vi "WindowPosition.vi"(4 "Komunikat":refnum<vi>, 6 "WindowHandler":refnum<vi>, 8 "error in (no error)":errorcluster, 9 "STOP":refnum<vi>, 10 "Tab":refnum<vi>, 11 "VI in":refnum<vi>) -> (0 "error out":errorcluster)   [LabVIEW 2019]
uses:
  <vilib>/Utility/miscctls.llb/LVRectTypeDef.ctl
  <vilib>/Utility/miscctls.llb/LVPointTypeDef.ctl
  <vilib>/Utility/miscctls.llb/LVBoundsTypeDef.ctl
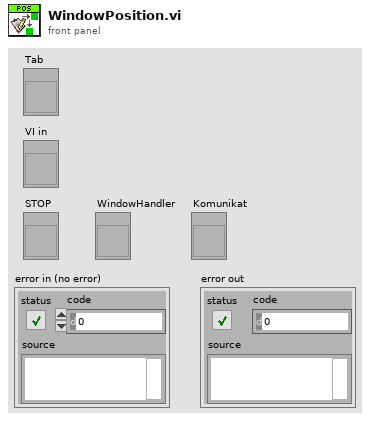
[diagram p1: front panel]
types:
  T1 = typedef "LVBoundsTypeDef.ctl" = cluster{"Width":u32, "Height":u32}
  T2 = typedef "LVPointTypeDef.ctl" = cluster{"Horizontal":i16, "Vertical":i16}
  T3 = typedef "LVRectTypeDef.ctl" = cluster{"Left":i16, "Top":i16, "Right":i16, "Bottom":i16}
  T4 = cluster{"Left":dbl, "Top":dbl, "Right":dbl, "Bottom":dbl}
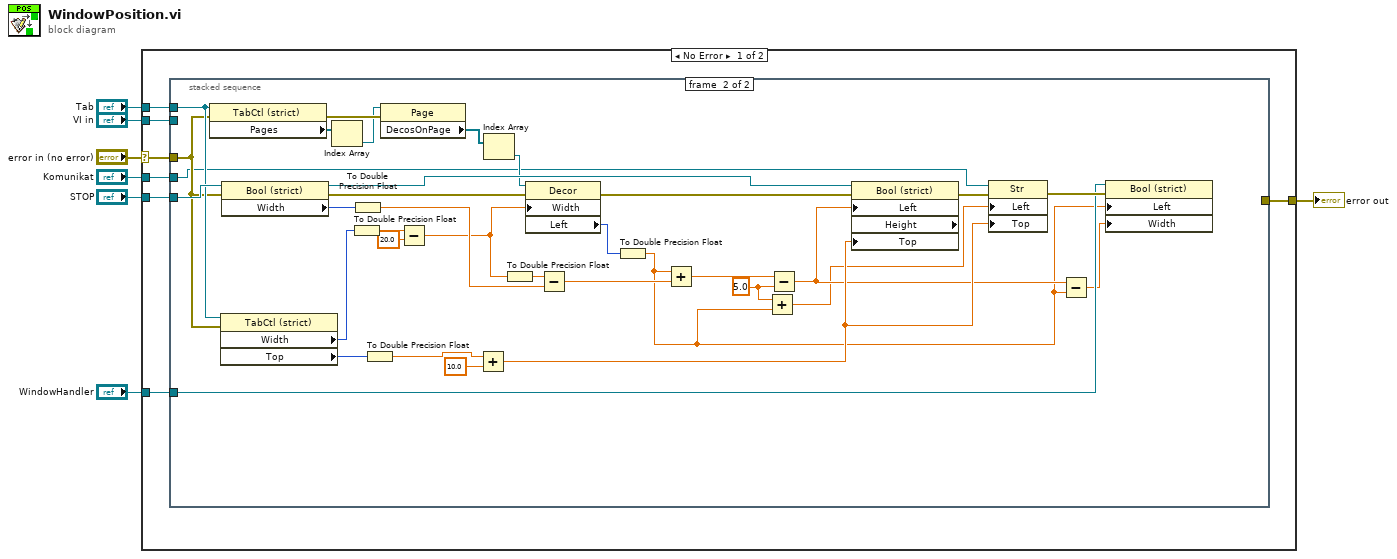
[diagram p0: block diagram]
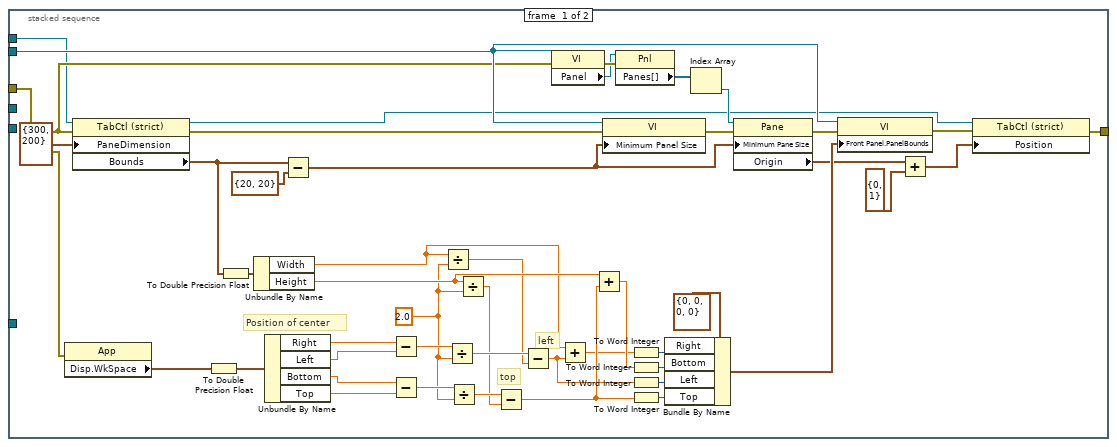
[diagram p2: hidden frame]
diagram:
  n1 = case shown="No Error" "error in (no error)" {
    selector: "error in (no error)" -> [w11 w95]
    tunnel: [w14 w95] -> w7
    tunnel: "Tab" -> [w13 _]
    tunnel: "VI in" -> [w12 _]
    tunnel: "STOP" -> [w10 _]
    tunnel: "Komunikat" -> [w9 _]
    tunnel: "WindowHandler" -> [w8 _]
    frame No Error {
      n2 = stacked-sequence {
        tunnel: [w60 _] -> w14
        tunnel: w13 -> [w17 w85]
        tunnel: w12 -> [w28 _]
        tunnel: w11 -> [w20 w84]
        tunnel: w10 -> [_ w86]
        tunnel: w9 -> [_ w82]
        tunnel: w8 -> [_ w65]
        frame #0 {
          w35 = 2.0
          # "Position of center"
          # "left"
          # "top"
          n3 = property class="App"(error in=w20) -> ("Disp.WkSpace"=w22:T3)  [unwired: 1 in, 2 out]
          n4 = property class="TabCtl (strict)"(reference=w17, error in=w20, "PaneDimension"=T1 {"Width"=300, "Height"=200} ("Tab Control Pane Dimension")) -> (reference out=w19:refnum<vi>, error out=w18:errorcluster, "Bounds"=w15:T1)
          n5 = To Double Precision Float(number=w22) -> (double precision float=w46:T4)
          n6 = To Double Precision Float(number=w15) -> (double precision float=w52:cluster{"Width":dbl, "Height":dbl})
          n7 = Unbundle By Name(w52) -> ("Width"=w34:dbl, "Height"=w54:dbl)
          n8 = Unbundle By Name(w46) -> ("Right"=w42:dbl, "Left"=w43:dbl, "Bottom"=w44:dbl, "Top"=w45:dbl)
          n9 = Subtract(x=w15, y=T2 {"Horizontal"=20, "Vertical"=20} ("Minimum Pane Size")) -> (x-y=w59:T1)
          n10 = Subtract(x=w42, y=w43) -> (x-y=w47:dbl)
          n11 = Subtract(x=w44, y=w45) -> (x-y=w48:dbl)
          n12 = Divide(x=w34, y=w35) -> (x/y=w33:dbl)
          n13 = Divide(x=w47, y=w35) -> (x/y=w36:dbl)
          n14 = Divide(x=w48, y=w35) -> (x/y=w37:dbl)
          n15 = Divide(x=w54, y=w35) -> (x/y=w32:dbl)
          n16 = Subtract(x=w37, y=w32) -> (x-y=w41:dbl)
          n17 = Subtract(x=w36, y=w33) -> (x-y=w40:dbl)
          n18 = property class="VI"(reference=w28, error in=w20) -> (error out=w57:errorcluster, "Panel"=w55:refnum<vi>)  [unwired: 1 out]
          n19 = Add(x=w34, y=w40) -> (x+y=w38:dbl)
          n20 = Add(x=w54, y=w41) -> (x+y=w39:dbl)
          n21 = property class="VI"(reference=w28, error in=w18, "Minimum Panel Size"=w59) -> (error out=w30:errorcluster)  [unwired: 1 out]
          n22 = property class="Pnl"(reference=w55, error in=w57) -> ("Panes[]"=w56:refnum<vi>[])  [unwired: 2 out]
          n23 = To Word Integer(number=w38) -> (16bit integer=w49:i16)
          n24 = To Word Integer(number=w39) -> (16bit integer=w51:i16)
          n25 = To Word Integer(number=w40) -> (16bit integer=w50:i16)
          n26 = To Word Integer(number=w41) -> (16bit integer=w53:i16)
          n27 = Bundle By Name(cluster=T3 {"Left"=0, "Top"=0, "Right"=0, "Bottom"=0} ("Front Panel Window:Panel Bounds"), "Right"=w49, "Bottom"=w51, "Left"=w50, "Top"=w53) -> (w27:T3)
          n28 = Index Array(array=w56) -> (element=w58:refnum<vi>)  [unwired: 1 in]
          n29 = property class="Pane"(reference=w58, error in=w30, "Minimum Pane Size"=w59) -> (error out=w29:errorcluster, "Origin"=w26:T2)  [unwired: 1 out]
          n30 = property class="VI"(reference=w28, error in=w29, "Front Panel.PanelBounds"=w27) -> (error out=w24:errorcluster)  [unwired: 1 out]
          n31 = Add(x=w26, y=T2 {"Horizontal"=0, "Vertical"=1}) -> (x+y=w25:T2)
          n32 = property class="TabCtl (strict)"(reference=w19, error in=w24, "Position"=w25) -> (error out=w60:errorcluster)  [unwired: 1 out]
        }
        frame #1 {
          w79 = 5.0 ("y")
          n33 = property class="TabCtl (strict)"(reference=w85, error in=w84) -> (error out=w90:errorcluster, "Pages"=w89:refnum<vi>[])  [unwired: 1 out]
          n34 = property class="TabCtl (strict)"(reference=w85, error in=w84) -> ("Width"=w71:u32, "Top"=w72:i32)  [unwired: 2 out]
          n35 = property class="Bool (strict)"(reference=w86, error in=w84) -> (reference out=w93:refnum<vi>, error out=w94:errorcluster, "Width"=w77:u32)
          n36 = Index Array(array=w89) -> (element=w88:refnum<vi>)  [unwired: 1 in]
          n37 = To Double Precision Float(number=w71) -> (double precision float=w70:dbl)
          n38 = To Double Precision Float(number=w77) -> (double precision float=w76:dbl)
          n39 = To Double Precision Float(number=w72) -> (double precision float=w73:dbl)
          n40 = property on="Property Node" class="Page"(reference=w88, error in=w90) -> ("DecosOnPage"=w91:refnum<vi>[])  [unwired: 2 out]
          n41 = Subtract(x=w70, y=20.0) -> (x-y=w68:dbl)
          n42 = Add(x=w73, y=10.0) -> (x+y=w80:dbl)
          n43 = Index Array(array=w91) -> (element=w87:refnum<vi>)  [unwired: 1 in]
          n44 = To Double Precision Float(number=w68) -> (double precision float=w75:dbl)
          n45 = property class="Decor"(reference=w87, error in=w94, "Width"=w68) -> (error out=w92:errorcluster, "Left"=w74:i32)  [unwired: 1 out]
          n46 = Subtract(x=w75, y=w76) -> (x-y=w67:dbl)
          n47 = To Double Precision Float(number=w74) -> (double precision float=w61:dbl)
          n48 = Add(x=w61, y=w67) -> (x+y=w83:dbl)
          n49 = Add(x=w79, y=w61) -> (x+y=w62:dbl)
          n50 = Subtract(x=w83, y=w79) -> (x-y=w64:dbl)
          n51 = property class="Bool (strict)" props=["Left", "Height", "Top"](reference=w93, error in=w92, "Left"=w64, "Top"=w80) -> (error out=w81:errorcluster)  [unwired: 2 out]
          n52 = property class="Str"(reference=w82, error in=w81, "Left"=w62, "Top"=w80) -> (error out=w66:errorcluster)  [unwired: 1 out]
          n53 = Subtract(x=w64, y=w61) -> (x-y=w63:dbl)
          n54 = property class="Bool (strict)"(reference=w65, error in=w66, "Left"=w61, "Width"=w63) -> ()  [unwired: 2 out]
        }
      }
    }
    frame Error {
    }
  }
  "error out" <- w7
